vi "Object in Elevator.vi"() -> (3 "Boolean":bool)   [LabVIEW 2014]
uses:
  Elevator Command.ctl
  Robot Global Data.vi
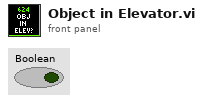
[diagram p1: front panel]
types:
  T1 = typedef "Elevator Command.ctl" = enum16{"Idle", "Load 1", "Load 2", "Load 3", "Drop Stack", "Eject Stack", "Load Trashcan"}
  T2 = typedef "Elevator Control Command.ctl" = cluster{"Command":T1, "Manual Motor Out":dbl, "Manual Eject Piston":bool, "Mode":T3, "Override Limits":bool, "Manual Stabilizer":bool, "Manual Finger":bool, "Load from Step?":bool, "Store Trashcan?":bool}
  T3 = typedef "Elevator Mode.ctl" = enum16{"Manual", "Safe", "Auto"}
  T4 = typedef "Dashboard Control Data.ctl" = cluster{"Cam Exposure":dbl, "Go to angle":dbl, "Steer PID Gains":cluster{"proportional gain (Kc)":dbl, "integral time (Ti, min)":dbl, "derivative time (Td, min)":dbl}, "Steer PID output Range":cluster{"output high":dbl, "output low":dbl}, "Pressure m \nValue":dbl, "Pressure b \nValue":dbl, "Strafe Timer\nWait":dbl, "Roller Command Cluster ":T5, "Elevator":T6, "Strafe Correct max steer":dbl, "IMU Enable":bool, "Encoder Control":T8, "IMU Controls":cluster{"Pitch Zero":dbl, "Roll Zero":dbl}}
  T5 = typedef "Roller Control.ctl" = cluster{"Intake Speed":dbl, "Turn In Speed":dbl, "Unload Speed":dbl, "Turn Out Speed":dbl, "Ping Align Tolerance":dbl, "Tote Range Threshold":dbl, "Right Pot 0":dbl, "Pot Threshold":dbl, "Left Pot 0":dbl, "Manual 0s?":bool, "Right Pot Scale":dbl, "Left Pot Scale":dbl, "0 wait time":i32, "Zero Pots":bool, "Min Elevator Height":dbl, "Eject Time":dbl, "Eject US Threshold":dbl}
  T6 = typedef "Elevator DB Control.ctl" = cluster{"PID Output Range":cluster{"output high":dbl, "output low":dbl}, "PID gains":cluster{"proportional gain (Kc)":dbl, "integral time (Ti, min)":dbl, "derivative time (Td, min)":dbl}, "Height Tolerance":sgl, " Encoder Constant":dbl, "Safe Mode Max Speed":sgl, "Eject Time":sgl, "Zeroing Speed":sgl, "Presets":T7, "Ping Detect Threshold":sgl, "Trashcan Detect Threshold":sgl}
  T7 = typedef "Elevator Presets.ctl" = cluster{"Hold Tote":sgl, "Hold Trashcan":sgl, "Pickup 2 w/ Tote":sgl, "Pickup 2 w/ Trashcan":sgl, "Pickup 3 w/ Tote":sgl, "Pickup 3 w/ Trashcan":sgl, "Bottom":sgl, "Pickup 1 w/ Tote":sgl, "Pickup Trashcan":sgl, "Pickup 1 w/ Trashcan":sgl, "Eject":sgl, "Hold 6":sgl, "Step add height":sgl, "Store Trashcan 3":sgl, "Store Trashcan 4":sgl, "Store Trashcan 5":sgl}
  T8 = typedef "Encoder Control.ctl" = cluster{"Left Tick Constant":dbl, "Right Tick Constant":dbl, "Center Tick Constant":dbl, "Reset?":bool, "Y Dist":cluster{"PID gains":cluster{"proportional gain (Kc)":dbl, "integral time (Ti, min)":dbl, "derivative time (Td, min)":dbl}, "output range":cluster{"output high":dbl, "output low":dbl}}, "X Dist":cluster{"PID gains":cluster{"proportional gain (Kc)":dbl, "integral time (Ti, min)":dbl, "derivative time (Td, min)":dbl}, "output range":cluster{"output high":dbl, "output low":dbl}}, "Y Stop Thresh":dbl, "Y Stop Speed":dbl, "X Stop Thresh":dbl, "X Stop Speed":dbl}
  T9 = typedef "Ultrasonic Indicators.ctl" = cluster{"Left Distance":dbl, "Right Distance":dbl, "Center Distance":dbl}
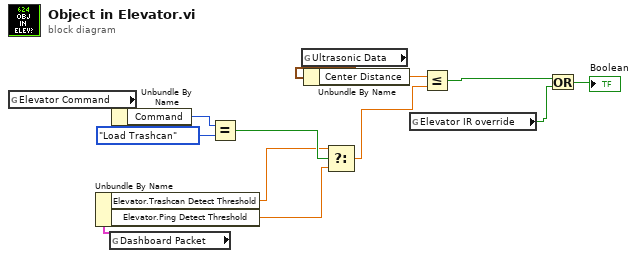
[diagram p0: block diagram]
diagram:
  n1 = global read "Robot Global Data.vi" "Elevator Command"() -> (w7:T2)
  n2 = global read "Robot Global Data.vi" "Dashboard Packet"() -> (w11:T4)
  n3 = Unbundle By Name(w11) -> ("Elevator.Trashcan Detect Threshold"=w2:sgl, "Elevator.Ping Detect Threshold"=w3:sgl)
  n4 = Unbundle By Name(w7) -> ("Command"=w6:T1)
  n5 = Equal?(x=w6, y=Elevator_Command."Load Trashcan") -> (x = y?=w4:bool)
  n6 = global read "Robot Global Data.vi" "Ultrasonic Data"() -> (w13:T9)
  n7 = Unbundle By Name(w13) -> ("Center Distance"=w12:dbl)
  n8 = Select(t=w2, s=w4, f=w3) -> (s? t:f=w1:sgl)
  n9 = global read "Robot Global Data.vi" "Elevator IR override"() -> (w10:bool)
  n10 = Less Or Equal?(x=w12, y=w1) -> (x <= y?=w9:bool)
  n11 = Or(x=w9, y=w10) -> (x .or. y?=→"Boolean":bool)
